vi "Beam Break control.vi"(11 "SRE ENUM":enum16{"Start", "Run", "End"}(ring)) -> (2 "2nd BB":bool=TRUE, 3 "1st BB":bool=TRUE)   [LabVIEW 2014]
uses:
  <vilib>/Rock Robotics/SystemInterfaces/DIO/FPGA_DIOChannel.ctl
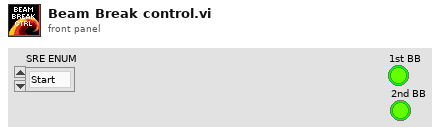
[diagram p1: front panel]
types:
  T1 = typedef "FPGA_DIOChannel.ctl" = enum8{"DIO 0", "DIO 1", "DIO 2", "DIO 3", "DIO 4", "DIO 5", "DIO 6", "DIO 7", "DIO 8", "DIO 9", "DIO MXP 0", "DIO MXP 1", "DIO MXP 2", "DIO MXP 3", "DIO MXP 4", "DIO MXP 5", "DIO MXP 6", "DIO MXP 7", "DIO MXP 8", "DIO MXP 9", "DIO MXP 10", "DIO MXP 11", "DIO MXP 12", "DIO MXP 13", "DIO MXP 14", "DIO MXP 15", "Invalid"}
  T2 = typedef "WPI_DigitalInputDevRef.ctl" = cluster{"DevStatus":errorcluster, "DIO Channel":T1, "Controller":T3}
  T3 = typedef "FPGA_TypedefDigitalModule.ctl" = enum16{"Controller 1"}
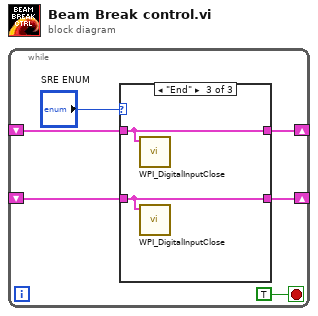
[diagram p0: block diagram]
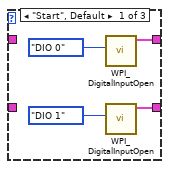
[diagram p2: hidden frame]
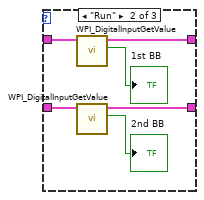
[diagram p3: hidden frame]
diagram:
  n1 = while {
    shift-right: [w5] -> _
    shift-left: _ -> [w2]
    shift-right: [w6] -> _
    shift-left: _ -> [w3]
    stop <- TRUE stop-if-true
    n2 = case shown="\"End\"" "SRE ENUM" {
      tunnel: [w10 w15 w17] -> w6
      tunnel: [w9 w14 w18] -> w5
      tunnel: w3 -> [_ w16 w17]
      tunnel: w2 -> [_ w13 w18]
      frame "Start", Default {
        n3 = call <vilib>:"WPI_DigitalInputOpen.vi"("DIO Channel"=FPGA_DIOChannel."DIO 0") -> ("DigitalInputDevRef"=w9:T2)  [unwired: 9 in, 1 out]
        n4 = call <vilib>:"WPI_DigitalInputOpen.vi"("DIO Channel"=FPGA_DIOChannel."DIO 1") -> ("DigitalInputDevRef"=w10:T2)  [unwired: 9 in, 1 out]
      }
      frame "Run" {
        n5 = call <vilib>:"WPI_DigitalInputGetValue.vi"("DigitalInputDevRef"=w13) -> ("Value"=→"1st BB":bool, "DigitalInputDevRef"=w14:T2)  [unwired: 8 in, 1 out]
        n6 = call <vilib>:"WPI_DigitalInputGetValue.vi"("DigitalInputDevRef"=w16) -> ("Value"=→"2nd BB":bool, "DigitalInputDevRef"=w15:T2)  [unwired: 8 in, 1 out]
      }
      frame "End" {
        n7 = call <vilib>:"WPI_DigitalInputClose.vi"("DigitalInputDevRef"=w18) -> ()  [unwired: 10 in, 1 out]
        n8 = call <vilib>:"WPI_DigitalInputClose.vi"("DigitalInputDevRef"=w17) -> ()  [unwired: 10 in, 1 out]
      }
    }
  }
